vi "save_file.vi"(5 "write header?":bool=TRUE, 7 "path":path, 8 "error in (no error)":errorcluster, 10 "ImageCollection in":refnum<class "ImageCollection.lvclass">, 11 "DataCollectionDL090215 in":refnum<class "DataCollectionDL090215.lvclass">) -> (0 "error out":errorcluster, 3 "DataCollectionDL090215 out":refnum<class "DataCollectionDL090215.lvclass">)   [LabVIEW 2010, in "DataCollectionDL090215.lvclass"]
uses:
  DataCollectionDL090215.lvclass
  common/classes/ImageCollection/ImageCollection/ImageCollection.lvclass
  common/classes/ImageCollection/ImageCollection/saving_parameters_cluster.ctl
  common/classes/Image/Image/target_format_enum.ctl
  common/classes/ImageCollection/ImageCollection/OME_parameters_cluster.ctl
  common/classes/ImageCollection/ImageCollection/dimension_order_enum.ctl
  common/classes/XMLElement/XMLElement/XMLElement.lvclass
  common/classes/ErrorController/ErrorController/class_data.vi
  common/classes/ErrorController/ErrorController/ErrorController.lvclass
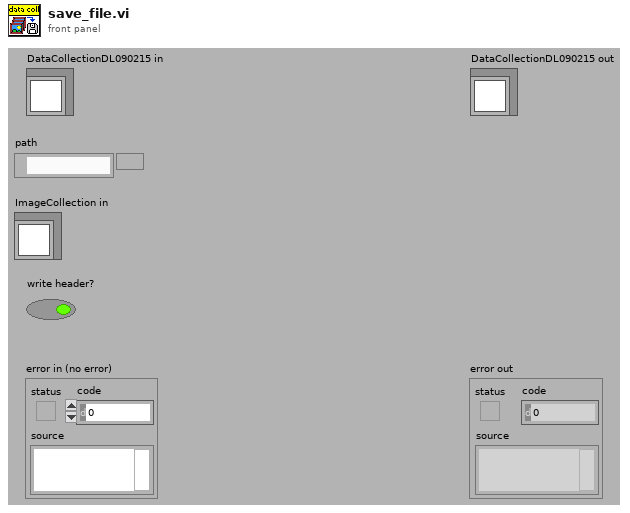
[diagram p1: front panel]
types:
  T1 = typedef "ImageCollection.lvclass/saving_parameters_cluster.ctl" = cluster{"write OME header?":bool, "save as list file?":bool, "force format?":T2, "multiplication factor":dbl, "offset":dbl}
  T2 = typedef "target_format_enum.ctl" = enum16{"don't force", "uint8", "uint16", "int16", "uint32", "int32", "single float"}
  T3 = typedef "dimension_order_enum.ctl" = enum16{"XYZCT", "XYZTC", "XYCTZ", "XYCZT", "XYTCZ", "XYTZC"}
  T4 = typedef "OME_parameters_cluster.ctl" = cluster{"image ID":string, "pixels ID":string, "dimension order":T3, "number of channels":i32}
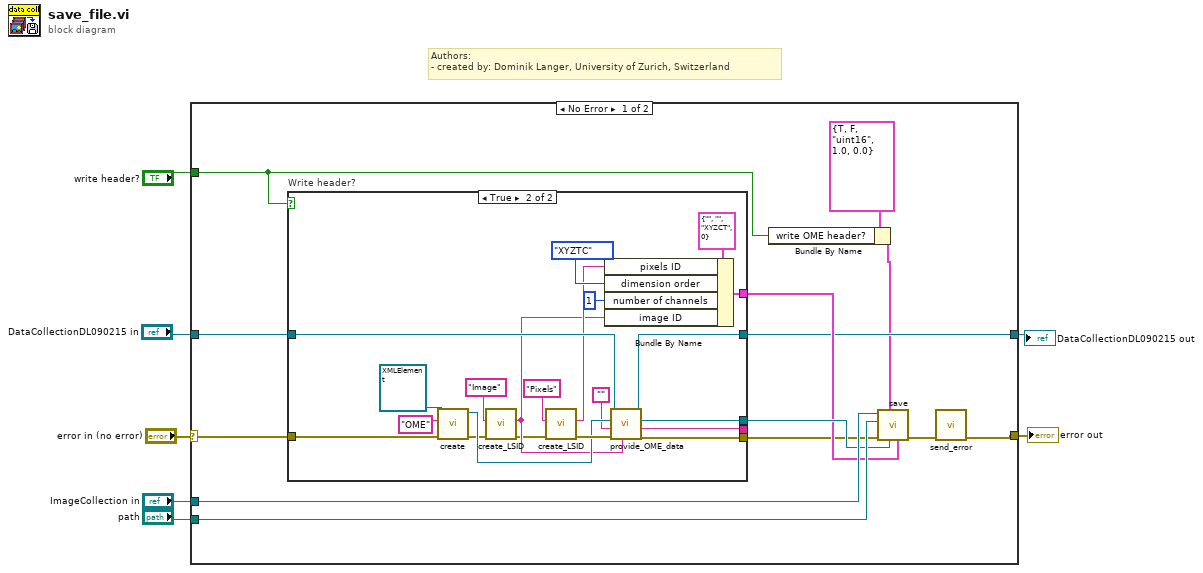
[diagram p0: block diagram]
diagram:
  # "Authors: \n- created by: Dominik Langer, University of Zurich, Switzerland"
  n1 = case shown="No Error" "error in (no error)" {
    selector: "error in (no error)" -> [w10 w45]
    tunnel: [w14 w45] -> w2
    tunnel: [w15 w44] -> w1
    tunnel: "DataCollectionDL090215 in" -> [w18 w44]
    tunnel: "path" -> [w20 _]
    tunnel: "ImageCollection in" -> [w19 _]
    tunnel: "write header?" -> [w11 _]
    frame No Error {
      n2 = case "Write header?" shown="True" w11 {
        tunnel: w18 -> [w21 w39]
        tunnel: [_ w37] -> w17
        tunnel: [_ w36] -> w16
        tunnel: [w22 w33] -> w9
        tunnel: w10 -> [w22 w32]
        tunnel: [w21 w34] -> w15
        tunnel: [_ w26] -> _
        frame False {
        }
        frame True {
          n3 = call "create.vi"("error in (no error)"=w32, "name"="OME", "XMLElement in"=refnum<class "XMLElement.lvclass"> refnum ("XMLElement.lvclass")) -> ("error out"=w24:errorcluster, "XMLElement out"=w31:refnum<class "XMLElement.lvclass">)  [unwired: 7 in]
          n4 = call "create_LSID.vi"("error in (no error)"=w24, "namespace"="Image") -> ("error out"=w25:errorcluster, "LSID"=w28:string)  [unwired: 8 in]
          n5 = call "create_LSID.vi"("error in (no error)"=w25, "namespace"="Pixels") -> ("error out"=w35:errorcluster, "LSID"=w38:string)  [unwired: 8 in]
          n6 = Bundle By Name(cluster=T4 {"image ID"="", "pixels ID"="", "dimension order"=enum."XYZCT", "number of channels"=0} ("OME parameters"), "pixels ID"=w38, "dimension order"=dimension_order_enum."XYZTC", "number of channels"=1, "image ID"=w28) -> (w36:T4)
          n7 = call-dynamic "provide_OME_data.vi"("image ID"=w28, "error in (no error)"=w35, "structuredAttribute string in"="", "OME element in"=w31, "DataCollectionDL091104Scaffold in"=w39) -> ("error out"=w33:errorcluster, "structuredAttribute string out"=w26:string, "OME element out"=w37:refnum<class "XMLElement.lvclass">, "DataCollectionDL091104Scaffold out"=w34:refnum<class "DataCollectionDL090215.lvclass">)  [unwired: 3 in]
        }
      }
      n8 = Bundle By Name(cluster=T1 {"write OME header?"=TRUE, "save as list file?"=FALSE, "force format?"=enum."uint16", "multiplication factor"=1.0, "offset"=0.0} ("saving parameters"), "write OME header?"=w11) -> (w12:T1)
      n9 = call "save.vi"("OME parameters"=w16, "OME XMLElement"=w17, "saving parameters"=w12, "error in (no error)"=w9, "path"=w20, "ImageCollection in"=w19) -> ("error out"=w8:errorcluster)  [unwired: 1 in, 4 out]
      n10 = call "send_error.vi"("error in (no error)"=w8) -> ("error out"=w14:errorcluster)  [unwired: 10 in]
    }
    frame Error {
    }
  }
  "error out" <- w2
  "DataCollectionDL090215 out" <- w1
